vi "Print Summary.vi"(8 "error in (no error)":errorcluster, 11 "Serializable Account in":refnum<class "Serializable Account.lvclass">) -> (0 "error out":errorcluster, 2 "Summary":string, 3 "Serializable Account out":refnum<class "Serializable Account.lvclass">)   [LabVIEW 2017, in "Serializable Account.lvclass"]
uses:
  Serializable Account.lvclass
  Serializable Account.lvclass/Serializable Account.ctl
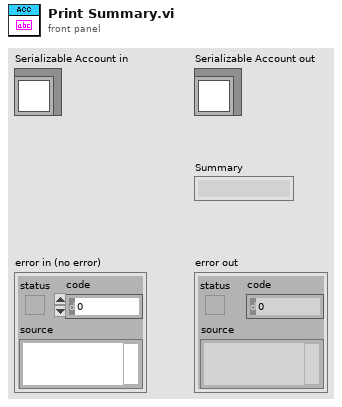
[diagram p1: front panel]
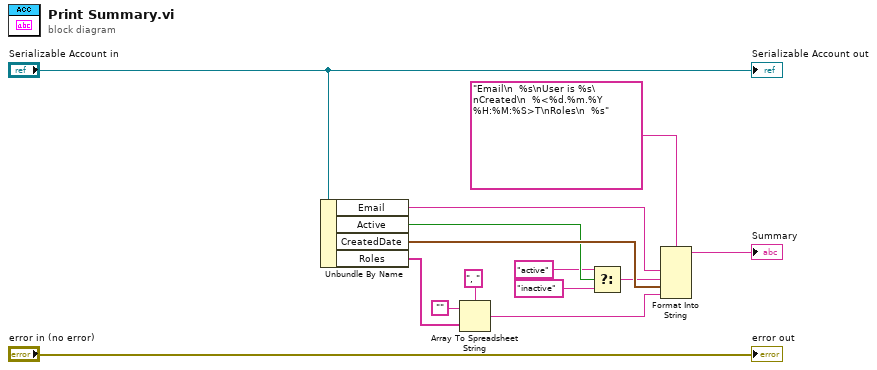
[diagram p0: block diagram]
diagram:
  n1 = Unbundle By Name("Serializable Account in") -> ("Email"=w7:string, "Active"=w8:bool, "CreatedDate"=w9:timestamp, "Roles"=w12:string[])
  n2 = Array To Spreadsheet String(delimiter (Tab)=", ", array=w12, 3:"") -> (spreadsheet string=w10:string)
  n3 = Select(t="active", s=w8, f="inactive") -> (s? t:f=w5:string)
  n4 = Format Into String(format string="Email\n  %s\nUser is %s\nCreated\n  %<%d.%m.%Y %H:%M:%S>T\nRoles\n  %s", w7, w5, w9, w10) -> (resulting string=→"Summary":string)  [unwired: 2 in, 1 out]
  "error out" <- "error in (no error)"
  "Serializable Account out" <- "Serializable Account in"
